vi "工件信息输入_子VI.vi"(8 "错误常量":errorcluster) -> (0 "错误常量out":errorcluster, 1 "产品规格":cluster{"产品长度（周长）（mm）":dbl, "产品宽度（母线长）（mm）":dbl}, 3 "图像分辨率":T1)   [LabVIEW 2018]
panel:
  in  "停止按钮":bool
  in  "产品宽度（母线长）（mm）":dbl format="%#_13g"
  in  "产品长度（周长）（mm）":dbl format="%#_13g"
  in  "图像Y向分辨率（mm/像素）":dbl=1.0 format="%#_13g"
  in  "图像X向分辨率（mm/像素）":dbl=1.0 format="%#_13g"
  # "图像及工件参数输入"
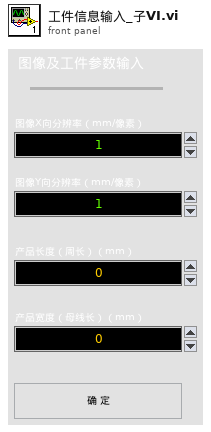
[diagram p1: front panel]
types:
  T1 = cluster{"图像X向分辨率（mm/像素）":dbl, "图像Y向分辨率（mm/像素）":dbl}
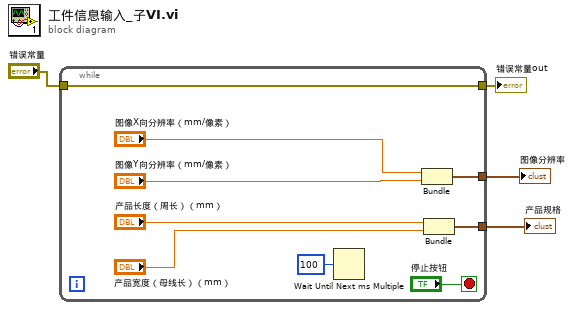
[diagram p0: block diagram]
diagram:
  n1 = while {
    tunnel: [w13] -> w4
    tunnel: [w12] -> w3
    tunnel: "错误常量" -> [w5]
    tunnel: [w5] -> w1
    stop <- "停止按钮" stop-if-true
    n2 = Wait Until Next ms Multiple(millisecond multiple=u32 100 ("毫秒倍数")) -> ()  [unwired: 1 out]
    n3 = Bundle("图像X向分辨率（mm/像素）"="图像X向分辨率（mm/像素）", "图像Y向分辨率（mm/像素）"="图像Y向分辨率（mm/像素）") -> (w13:T1)  [unwired: 1 in]
    n4 = Bundle("产品长度（周长）（mm）"="产品长度（周长）（mm）", "产品宽度（母线长）（mm）"="产品宽度（母线长）（mm）") -> (w12:cluster{"产品长度（周长）（mm）":dbl, "产品宽度（母线长）（mm）":dbl})  [unwired: 1 in]
  }
  "图像分辨率" <- w4
  "产品规格" <- w3
  "错误常量out" <- w1
